vi "Read UnhandledShutdown.vi"(8 "error in (no error)":errorcluster, 11 "Attribute.StartupBehavior in":refnum<class "Attribute.ErrorHandling.lvclass">) -> (0 "error out":errorcluster, 2 "Shutdown on Unhandled Error":bool, 3 "Attribute.StartupBehavior out":refnum<class "Attribute.ErrorHandling.lvclass">)   [LabVIEW 2013, in "Attribute.ErrorHandling.lvclass"]
uses:
  Attribute.ErrorHandling.lvclass
  Attribute.ErrorHandling.lvclass/Attribute.ErrorHandling.ctl
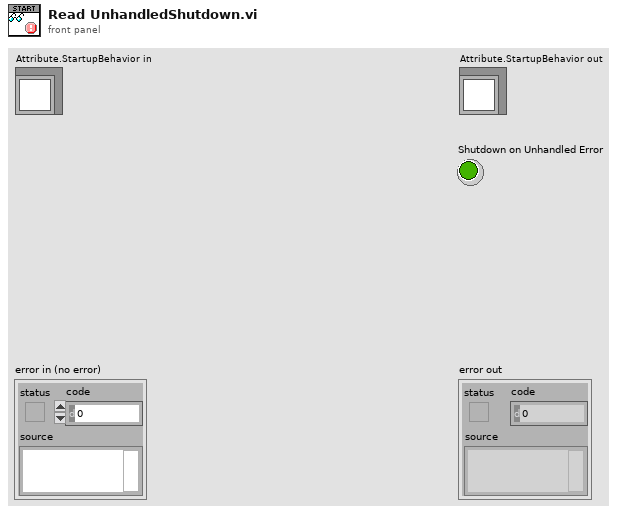
[diagram p1: front panel]
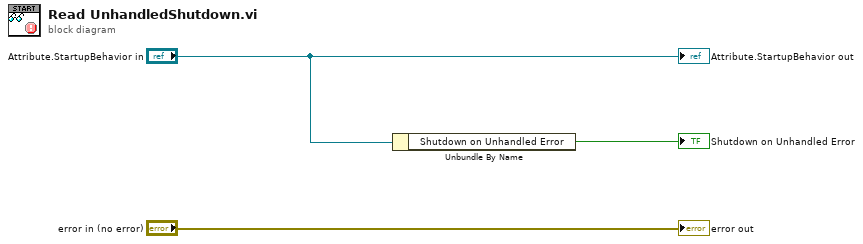
[diagram p0: block diagram]
diagram:
  n1 = Unbundle By Name("Attribute.StartupBehavior in") -> ("Shutdown on Unhandled Error"=→"Shutdown on Unhandled Error":bool)
  "error out" <- "error in (no error)"
  "Attribute.StartupBehavior out" <- "Attribute.StartupBehavior in"
